vi "SubtractionClassTest.vi"(8 "error in (no error)":errorcluster) -> (0 "error out":errorcluster)   [LabVIEW 2023, in "TestLib.lvlib"]
doc: "This VI tests the subtract method class with some random test cases using caraya."
uses:
  TestLib.lvlib
  Typedef/TestCaseSampleIO.ctl
  Arithmetic/Arithmetic.lvclass
  <vilib>/addons/_JKI Toolkits/Caraya/classes/Assert/Assert Equal Value_Variant.vi
  <vilib>/addons/_JKI Toolkits/Caraya/classes/Test/Test.lvclass
  <vilib>/addons/_JKI Toolkits/Caraya/classes/Assert/Assert.lvclass
panel:
  # "SUBTRACTION CLASS TEST VI"
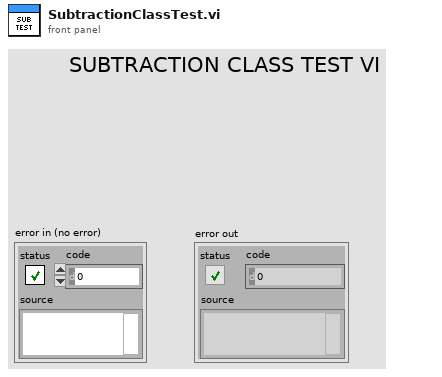
[diagram p1: front panel]
types:
  T1 = typedef "TestCaseSampleIO.ctl" = cluster{"Input1":dbl, "Input2":dbl, "Output":dbl}
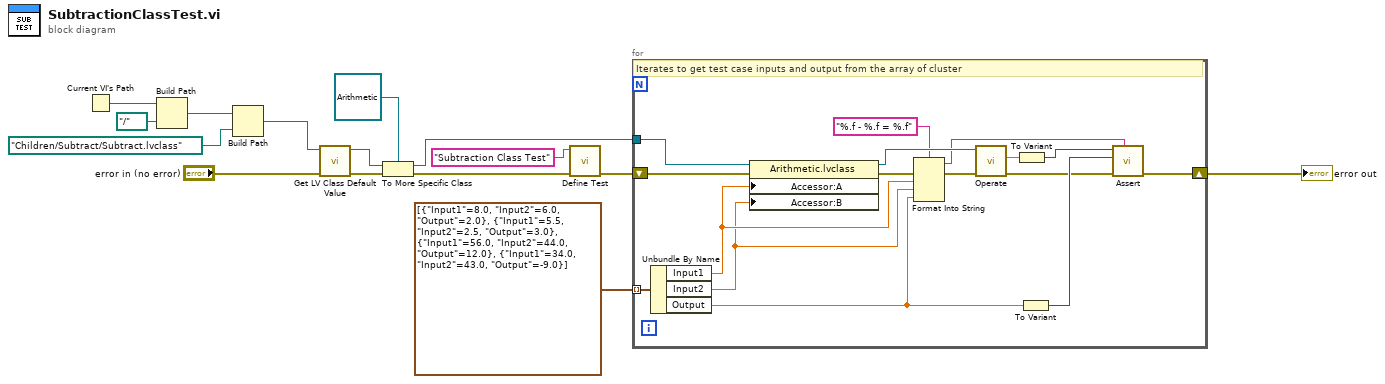
[diagram p0: block diagram]
diagram:
  n1 = Current VI's Path() -> (path=w11:path)
  n2 = Build Path(base path=w11, name or relative path=path "../..") -> (appended path=w9:path)
  n3 = Build Path(base path=w9, name or relative path=path "Children/Subtract/Subtract.lvclass") -> (appended path=w7:path)
  n4 = call <vilib>:"Get LV Class Default Value.vi"("error in (no error)"="error in (no error)", "class path"=w7) -> ("error out"=w2:errorcluster, "object"=w6:refnum<class>)  [unwired: 8 in]
  n5 = To More Specific Class(target class=refnum<class "Arithmetic.lvclass"> refnum ("Arithmetic.lvclass"), reference=w6, error in=w2) -> (specific class reference=w4:refnum<class "Arithmetic.lvclass">, error out=w1:errorcluster)
  n6 = call <vilib>:"Define Test.vi"("error in (no error)"=w1, "Label (VI Title)"="Subtraction Class Test") -> ("error out"=w15:errorcluster)  [unwired: 8 in, 1 out]
  n7 = for {
    tunnel: w4 -> [w31]
    shift-right: [w29] -> w13
    shift-left: w15 -> [w30]
    tunnel: T1[] [{"Input1"=8.0, "Input2"=6.0, "Output"=2.0}, {"Input1"=5.5, "Input2"=2.5, "Output"=3.0}, {"Input1"=56.0, "Input2"=44.0, "Output"=12.0}, {"Input1"=34.0, "Input2"=43.0, "Output"=-9.0}] -> [w28] mode=indexing
    # "Iterates to get test case inputs and output from the array of cluster"
    n8 = Unbundle By Name(w28) -> ("Input1"=w20:dbl, "Input2"=w19:dbl, "Output"=w18:dbl)
    n9 = property class="Arithmetic.lvclass"(reference=w31, error in=w30, "Accessor:A"=w20, "Accessor:B"=w19) -> (reference out=w24:refnum<class "Arithmetic.lvclass">, error out=w25:errorcluster)
    n10 = Format Into String(format string="%.f - %.f = %.f", error in=w25, w20, w19, w18) -> (resulting string=w16:string, error out=w21:errorcluster)  [unwired: 1 in]
    n11 = call-dynamic "Operate.vi"("error in (no error)"=w21, "Arithmetic in"=w24) -> ("error out"=w23:errorcluster, "C"=w22:dbl)  [unwired: 7 in, 1 out]
    n12 = To Variant(anything=w22) -> (Variant=w27:variant)
    n13 = To Variant(anything=w18) -> (Variant=w26:variant)
    n14 = call-poly <vilib>:"Assert.vi"("Label"=w16, "error in (no error)"=w23, "Y"=w26, "X"=w27) -> ("error out"=w29:errorcluster)  [unwired: 6 in, 1 out]
  }
  "error out" <- w13
